vi "To ICommunicate.vi"(8 "error in":errorcluster, 11 "LabVIEW Object":refnum<class>) -> (0 "error out":errorcluster, 3 "ICommunicate":refnum<class "ICommunicate.lvclass">)   [LabVIEW 2025]
uses:
  ICommunicate.lvclass
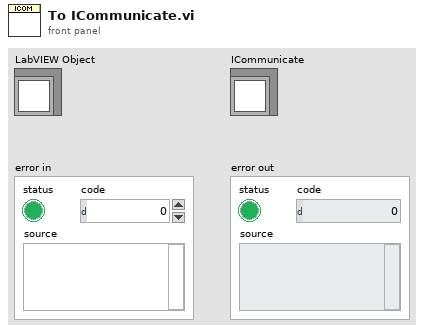
[diagram p1: front panel]
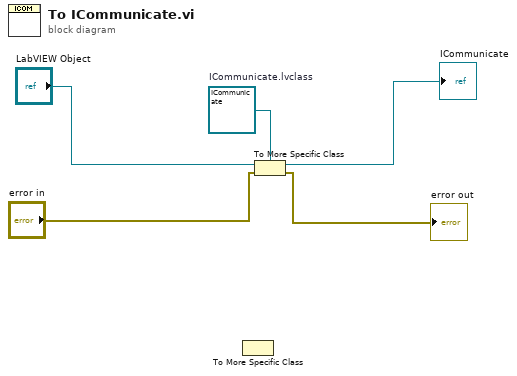
[diagram p0: block diagram]
diagram:
  w5 = refnum<class "ICommunicate.lvclass"> refnum  # ICommunicate.lvclass
  n1 = To More Specific Class() -> ()  [unwired: 3 in, 2 out]
  n2 = To More Specific Class(target class=w5, reference="LabVIEW Object", error in="error in") -> (specific class reference=→"ICommunicate":refnum<class "ICommunicate.lvclass">, error out=→"error out":errorcluster)
